vi "open_camera.vi"(6 "Number of Buffers":u32=10, 7 "OverwriteMode":u32(ring) items=["Get Oldest"=0, "Fail"=2, "Get Newest"=3], 8 "error in":errorcluster, 9 "VideoMode":u32=9, 10 "ValueDBL":dbl=50.0 format="%#_13g", 11 "Session In":T1="cam0") -> (0 "error out":errorcluster, 3 "Session Out":T1)   [LabVIEW 2019]
uses:
  <vilib>/userdefined/High Color/IMAQdx.ctl
  <vilib>/vision/driver/NI_Vision_Acquisition_Software.lvlib
  <resource>/objmgr/imaqdx.rc
panel:
  in  "ActiveAttribute":string="HardwareRequeueBufferListThreshold"
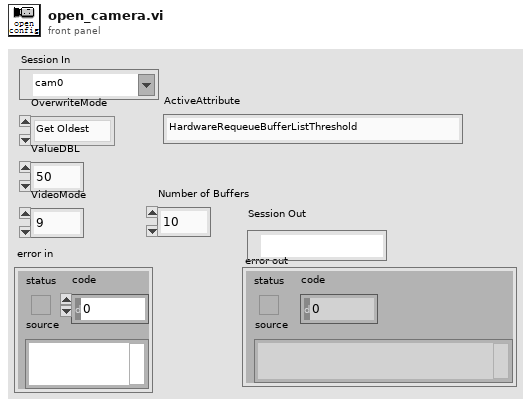
[diagram p1: front panel]
types:
  T1 = typedef "IMAQdx.ctl" = refnum<k21>
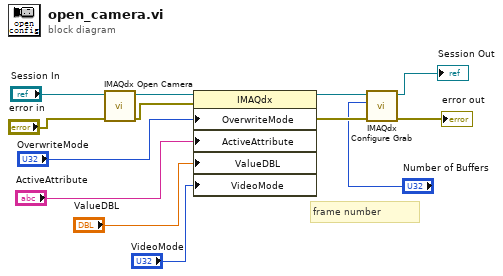
[diagram p0: block diagram]
diagram:
  # "frame number"
  n1 = call <vilib>:"IMAQdx Open Camera.vi"("error in"="error in", "Session In"="Session In") -> ("error out"=w1:errorcluster, "Session Out"=w2:T1)  [unwired: 8 in]
  n2 = property class="IMAQdx"(reference=w2, error in=w1, "OverwriteMode"="OverwriteMode", "ActiveAttribute"="ActiveAttribute", "ValueDBL"="ValueDBL", "VideoMode"="VideoMode") -> (reference out=w13:T1, error out=w12:errorcluster)
  n3 = call <vilib>:"IMAQdx Configure Grab.vi"("error in"=w12, "Number of Buffers"="Number of Buffers", "Session In"=w13) -> ("error out"=→"error out":errorcluster, "Session Out"=→"Session Out":T1)  [unwired: 7 in]
